vi "rename class.vi"(8 "error in":errorcluster, 9 "new name":string, 10 "class path":path, 11 "Application in":refnum<vi>) -> (0 "error out":errorcluster, 3 "New Library Path":path)   [LabVIEW 2013, in "TagBusProcessingPluginFeatureDecider.lvclass"]
uses:
  TagBusProcessingPluginFeatureDecider.lvclass
  <vilib>/Utility/EditLVLibs/Edit LVLibs.lvlib
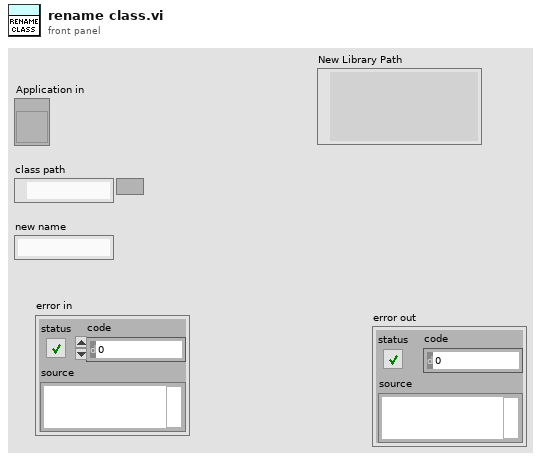
[diagram p1: front panel]
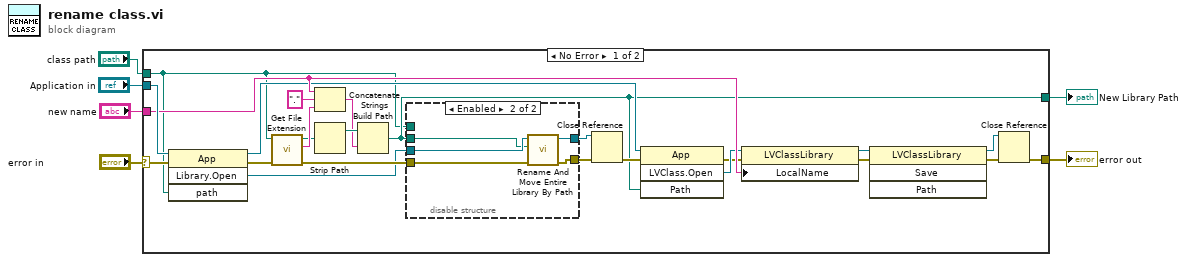
[diagram p0: block diagram]
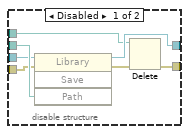
[diagram p2: hidden frame]
diagram:
  n1 = case shown="No Error" "error in" {
    selector: "error in" -> [w13 w43]
    tunnel: [w30 w43] -> w6
    tunnel: "Application in" -> [w27 _]
    tunnel: "class path" -> [w7 _]
    tunnel: "new name" -> [w23 _]
    tunnel: [w12 _] -> w2
    frame No Error {
      n2 = invoke class="App" method="Library.Open"(reference=w27, error in=w13, "path"=w7) -> (reference out=w18:refnum<vi>, error out=w26:errorcluster, "Open Library"=w9:refnum<vi>)  [unwired: 1 in, 1 out]
      n3 = call <vilib>:"Get File Extension.vi"("error in (no error)"=w26, "file"=w7) -> ("error out"=w11:errorcluster, "lowercase file extension"=w25:string, "dup file"=w22:path)  [unwired: 6 in, 1 out]
      n4 = Concatenate Strings(w23, "." ("string"), w25) -> (w20:string)
      n5 = Strip Path(path=w22) -> (stripped path=w21:path)  [unwired: 1 out]
      n6 = Build Path(base path=w21, name or relative path=w20) -> (appended path=w12:path)
      n7 = disable-structure shown="Enabled" {
        disable-tunnel: w12 -> [w36 w38]
        disable-tunnel: w11 -> [w35 w40]
        disable-tunnel: [w34 w41] -> w10
        disable-tunnel: w9 -> [w33 w39]
        disable-tunnel: [w32 w42] -> w8
        disable-tunnel: w7 -> [w31 _]
        frame Disabled {
          n8 = invoke class="Library" method="Save"(reference=w33, error in=w35, "Path"=w36) -> (reference out=w32:refnum<vi>, error out=w37:errorcluster)  [unwired: 1 in, 2 out]
          n9 = Delete(path (use dialog)=w31, error in=w37) -> (error out=w34:errorcluster)  [unwired: 3 in, 2 out]
        }
        frame Enabled {
          n10 = call <vilib>:"Rename And Move Entire Library By Path.vi"("error in (no error)"=w40, "New library path"=w38, "Library ref in"=w39) -> ("error out"=w41:errorcluster, "Library ref out"=w42:refnum<vi>)  [unwired: 7 in]
        }
      }
      n11 = Close Reference(reference=w8, error in (no error)=w10) -> (error out=w19:errorcluster)
      n12 = invoke class="App" method="LVClass.Open"(reference=w18, error in=w19, "Path"=w12) -> (error out=w16:errorcluster, "LVClass.Open"=w17:refnum<vi>)  [unwired: 1 in, 2 out]
      n13 = property class="LVClassLibrary"(reference=w17, error in=w16, "LocalName"=w23) -> (reference out=w29:refnum<vi>, error out=w28:errorcluster)
      n14 = invoke class="LVClassLibrary" method="Save"(reference=w29, error in=w28) -> (reference out=w14:refnum<vi>, error out=w15:errorcluster)  [unwired: 2 in, 2 out]
      n15 = Close Reference(reference=w14, error in (no error)=w15) -> (error out=w30:errorcluster)
    }
    frame Error {
    }
  }
  "error out" <- w6
  "New Library Path" <- w2
